vi "Configure DAQ channel.vi"(8 "error in (no error)":errorcluster, 10 "String":string, 11 "DAQ ID":i32) -> (0 "error out":errorcluster)   [LabVIEW 2025]
uses:
  Libraries/NI DAQ/NI DAQ.lvlib
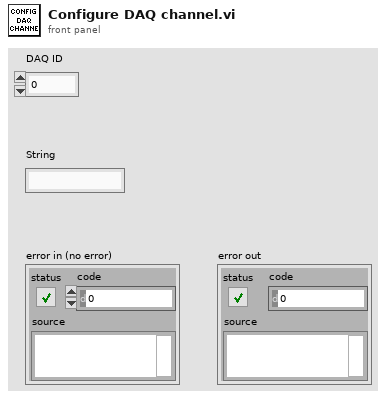
[diagram p1: front panel]
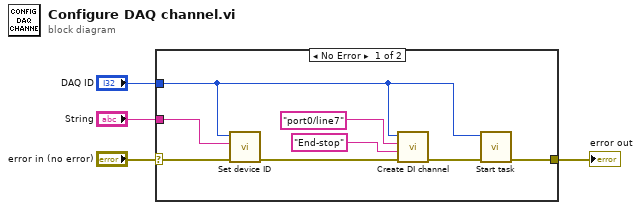
[diagram p0: block diagram]
diagram:
  n1 = case shown="No Error" "error in (no error)" {
    selector: "error in (no error)" -> [w12 w13]
    tunnel: "DAQ ID" -> [w11 _]
    tunnel: [w10 w13] -> w2
    tunnel: "String" -> [w5 _]
    frame No Error {
      n2 = call "Set device ID.vi"("error in"=w12, "Device ID"=w5, "Module ID"=w11) -> ("error out"=w6:errorcluster)  [unwired: 8 in]
      n3 = call "Create DI channel.vi"("error in"=w6, "Channel name"="End-stop", "Physical channel"="port0/line7", "Module ID"=w11) -> ("error out"=w9:errorcluster)  [unwired: 7 in]
      n4 = call "Start task.vi"("error in"=w9, "Module ID"=w11) -> ("error out"=w10:errorcluster)  [unwired: 9 in]
    }
    frame Error {
    }
  }
  "error out" <- w2
